vi "Scan Control View.vi"(10 "User Events in":refnum<class "User Events.lvclass">) -> ()   [LabVIEW 2016, in "HPMT_Views.lvlib"]
uses:
  HPMT_Views.lvlib
  User Events/User Events.lvclass
  Commands/Command Factory/Command Factory.lvclass
  User Events/User Events.lvclass/User Events.ctl
  Typedefs/TestSettings.ctl
  Typedefs/StateTypes.ctl
  Commands/Start Testing Command/Start Testing Command.lvclass
  Commands/Start Testing Command/Start Testing Command.lvclass/Start Testing Command.ctl
  Commands/Manual Mode Command/Manual Mode Command.lvclass
  Typedefs/HPMT_Typedefs.lvlib
panel:
  in  "Micron to Encoder Ratio":dbl=0.2442
  in  "Micron to Step Ratio":dbl=0.0607
  in  "Load Cell Sensitivity":dbl=1.079
  in  "Manual Mode":bool
  in  "Largest Strut Displacement":dbl=3.0
  in  "Breakaway Air Pressure":u16=120
  in  "Settling Time (secs)":u16=2
  in  "Data Points per Cycle":u16=20
  in  "Number of Cycles":u16=2
  in  "Test Angle":u16=90
  in  "Strut Number":string="1"
  in  "Notes":string
  in  "Operator":string="aclements"
  in  "Test Stand Serial Number":string="1"
  in  "StartTest":bool
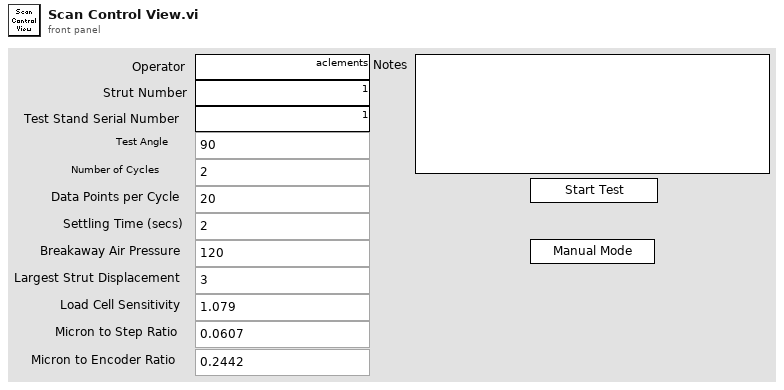
[diagram p1: front panel]
types:
  T1 = typedef "HPMT_Typedefs.lvlib/Publish Data Events.ctl" = cluster{"State":refnum<user-event>, "ErrorCode":refnum<user-event>, "Scan Progress":refnum<user-event>, "All Test Status":refnum<user-event>, "ActuatorData":refnum<user-event>, "Test Settings":refnum<user-event>, "Stop Constant Query":refnum<user-event>}
  T2 = typedef "HPMT_Typedefs.lvlib/Subscribe Data Events.ctl" = cluster{"Command":refnum<user-event>}
  T3 = cluster{"Event Registration Refnum":refnum<event-registration>}
  T4 = typedef "HPMT_Typedefs.lvlib/TestSettings.ctl" = cluster{"Operator":string, "Strut Number":string, "Test Stand Serial Number":string, "Notes":string, "Test Angle":u16, "Number of Cycles":u16, "Data Points per Cycle":u16, "Settling Time (secs)":u16, "Breakaway Air Pressure":u16, "Largest Strut Displacement":dbl, "Load Cell Sensitivity":dbl, "Micron to Step Ratio":dbl, "Micron to Encoder Ratio":dbl, "Software Version":string}
  T5 = typedef "HPMT_Typedefs.lvlib/StateTypes.ctl" = enum16{"Offline State", "Fault State", "Standby State", "Disabled State", "Enabled State", "Wait For User Input State", "Test Actuator State", "Manual State"}
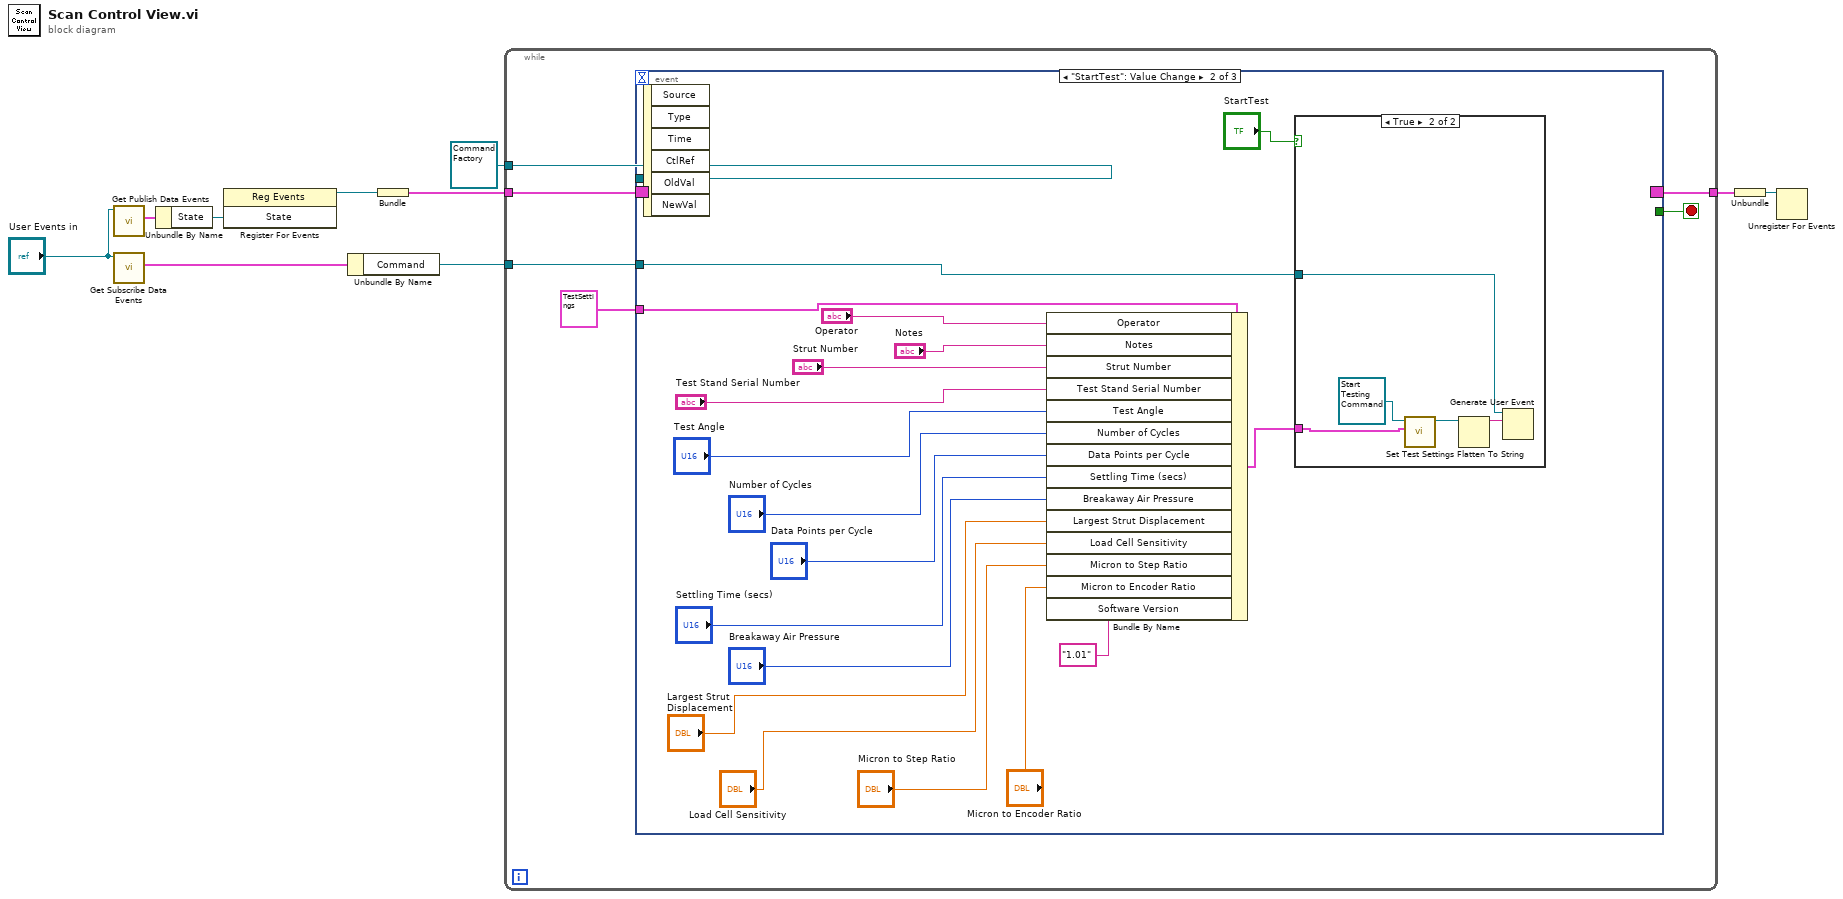
[diagram p0: block diagram]
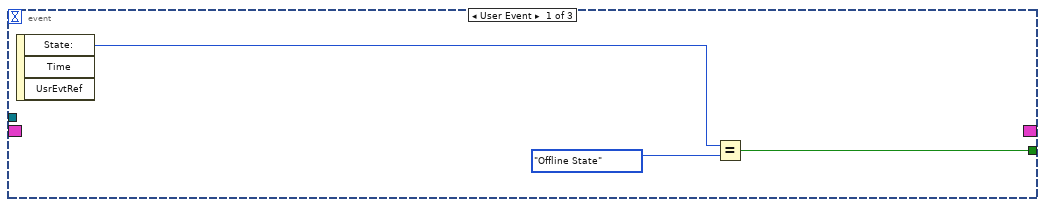
[diagram p2: hidden frame]
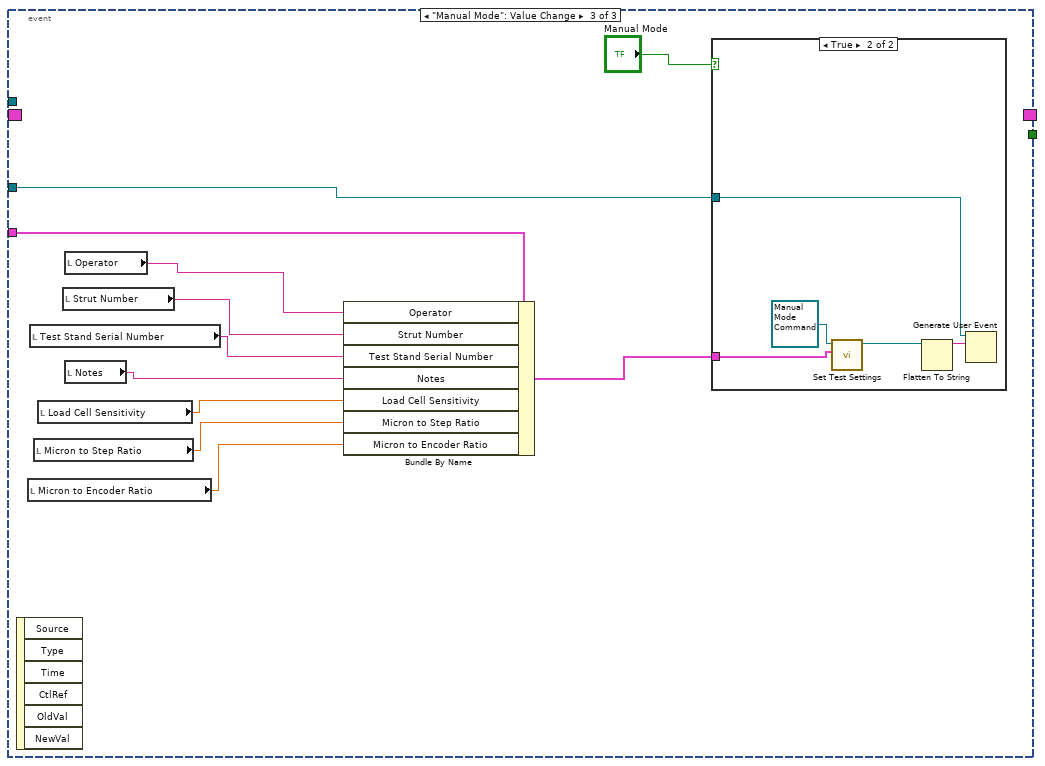
[diagram p4: hidden frame]
diagram:
  n1 = call "Get Publish Data Events.vi"("UserEvents in"="User Events in") -> ("Publish Data Events"=w10:T1)  [unwired: 9 in, 1 out]
  n2 = call "Get Subscribe Data Events.vi"("UserEvents in"="User Events in") -> ("Subscribe Data Events"=w4:T2)  [unwired: 9 in, 1 out]
  n3 = Unbundle By Name(w10) -> ("State"=w9:refnum<user-event>)
  n4 = register-events(w9) -> (reference out=w8:refnum<event-registration>)  [unwired: 2 in, 1 out]
  n5 = Unbundle By Name(w4) -> ("Command"=w2:refnum<user-event>)
  n6 = Bundle("Event Registration Refnum"=w8) -> (w5:T3)  [unwired: 1 in]
  n7 = while {
    tunnel: w5 -> [w16]
    tunnel: [w15] -> w6
    tunnel: w2 -> [w13]
    tunnel: refnum<class "Command Factory.lvclass"> refnum ("CommandFactory.lvclass") -> [w12]
    stop <- w14 stop-if-true
    n8 = event shown="[1] \"StartTest\": Value Change" {
      selector: w16 -> [_ _ _]
      dyn-events: [_ _ _] -> w15
      timeout: _ -> [_ _ _]
      tunnel: [w18 _ _] -> w14
      tunnel: w13 -> [_ w36 w52]
      tunnel: w12 -> [_ _ _]
      tunnel: T4 {"Operator"="", "Strut Number"="", "Test Stand Serial Number"="", "Notes"="", "Test Angle"=0, "Number of Cycles"=0, "Data Points per Cycle"=0, "Settling Time (secs)"=0, "Breakaway Air Pressure"=0, "Largest Strut Displacement"=0.0, "Load Cell Sensitivity"=0.0, "Micron to Step Ratio"=0.0, "Micron to Encoder Ratio"=0.04883, "Software Version"=""} ("Scan Settings") -> [_ w23 w51]
      event User Event {
        n9 = event-data() -> ("State:"=w17:T5)  [unwired: 1 in, 2 out]
        n10 = Equal?(x=w17, y=StateTypes."Offline State") -> (x = y?=w18:bool)
      }
      event "StartTest": Value Change {
        n11 = event-data() -> ()  [unwired: 1 in, 6 out]
        n12 = Bundle By Name(cluster=w23, "Operator"="Operator", "Notes"="Notes", "Strut Number"="Strut Number", "Test Stand Serial Number"="Test Stand Serial Number", "Test Angle"="Test Angle", "Number of Cycles"="Number of Cycles", "Data Points per Cycle"="Data Points per Cycle", "Settling Time (secs)"="Settling Time (secs)", "Breakaway Air Pressure"="Breakaway Air Pressure", "Largest Strut Displacement"="Largest Strut Displacement", "Load Cell Sensitivity"="Load Cell Sensitivity", "Micron to Step Ratio"="Micron to Step Ratio", "Micron to Encoder Ratio"="Micron to Encoder Ratio", "Software Version"="1.01") -> (w24:T4)
        n13 = case shown="True" "StartTest" {
          tunnel: w36 -> [_ w42]
          tunnel: w24 -> [_ w38]
          frame False {
          }
          frame True {
            n14 = call "Set Test Settings.vi"("Test Settings"=w38, "Start Closed Loop Scan Command in"=refnum<class "Start Testing Command.lvclass"> refnum ("Start Scan Command.lvclass")) -> ("Start Closed Loop Scan Command out"=w40:refnum<class "Start Testing Command.lvclass">)  [unwired: 9 in]
            n15 = Flatten To String(anything=w40) -> (data string=w41:string)  [unwired: 3 in, 2 out]
            n16 = Generate User Event(user event=w42, event data cluster=w41) -> ()  [unwired: 2 in, 2 out]
          }
        }
      }
      event "Manual Mode": Value Change {
        n17 = event-data() -> ()  [unwired: 1 in, 6 out]
        n18 = local read "Micron to Encoder Ratio"() -> (w43:dbl)
        n19 = local read "Test Stand Serial Number"() -> (w47:string)
        n20 = local read "Micron to Step Ratio"() -> (w44:dbl)
        n21 = local read "Load Cell Sensitivity"() -> (w45:dbl)
        n22 = local read "Strut Number"() -> (w48:string)
        n23 = local read "Operator"() -> (w49:string)
        n24 = local read "Notes"() -> (w46:string)
        n25 = Bundle By Name(cluster=w51, "Operator"=w49, "Strut Number"=w48, "Test Stand Serial Number"=w47, "Notes"=w46, "Load Cell Sensitivity"=w45, "Micron to Step Ratio"=w44, "Micron to Encoder Ratio"=w43) -> (w50:T4)
        n26 = case shown="True" "Manual Mode" {
          tunnel: w52 -> [_ w56]
          tunnel: w50 -> [_ w54]
          frame False {
          }
          frame True {
            n27 = call "Set Test Settings.vi"("Test Settings"=w54, "Manual Mode Command in"=refnum<class "Manual Mode Command.lvclass"> refnum ("Manual Mode Command.lvclass")) -> ("Manual Mode Command out"=w57:refnum<class "Manual Mode Command.lvclass">)  [unwired: 9 in]
            n28 = Flatten To String(anything=w57) -> (data string=w55:string)  [unwired: 3 in, 2 out]
            n29 = Generate User Event(user event=w56, event data cluster=w55) -> ()  [unwired: 2 in, 2 out]
          }
        }
      }
    }
  }
  n30 = Unbundle(w6) -> ("Event Registration Refnum"=w7:refnum<event-registration>)
  n31 = Unregister For Events(event registration refnum=w7) -> ()  [unwired: 1 in, 1 out]
